vi "Init.vi"(8 "error in (no error)":errorcluster, 11 "reference in":refnum<class "PSU_Keysight_34951A.lvclass">) -> (0 "error out":errorcluster, 3 "reference out":refnum<class "PSU_Keysight_34951A.lvclass">)   [LabVIEW 2022 SP3, in "PSU_Keysight_34951A.lvlib" / "PSU_Keysight_34951A.lvclass"]
uses:
  PSU_Keysight_34951A.lvclass
  Components/PSU_Base.lvlibp/PSU_Base.lvclass
  Components/ViPER.lvlibp/ViPER.lvclass
  C:/Projects/Medulla/ViPER/Examples/Flux_Capacitor_Tester/Components/ViPER.lvlibp/ViPER.lvclass
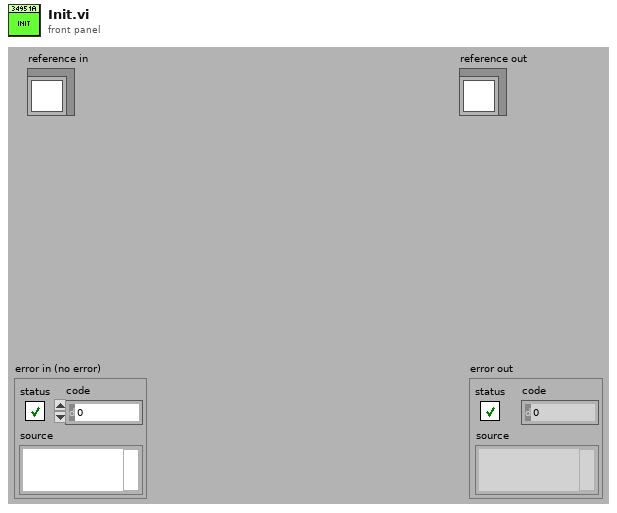
[diagram p1: front panel]
types:
  T1 = typedef "PSU_Keysight_34951A.lvlib/PSU_Keysight_34951A.lvclass/ObjectAttributes.ctl" = cluster{"Config":T2, "VISA res":refnum<visa-resource-name>, "Enabled":bool[], "V":dbl[], "I":dbl[], "Source Type":enum16{"Voltage", "Current"}[]}
  T2 = typedef "PSU_Keysight_34951A.lvlib/PSU_Keysight_34951A.lvclass/Config.ctl" = cluster{"VISA":refnum<visa-resource-name>, "Slot":i32}
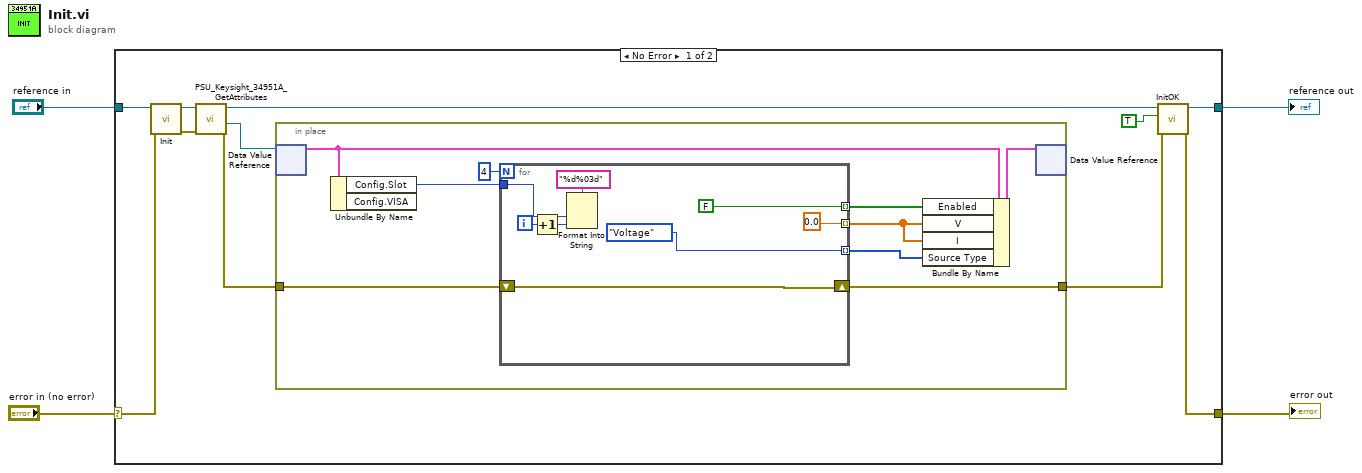
[diagram p0: block diagram]
diagram:
  n1 = case shown="No Error" "error in (no error)" {
    selector: "error in (no error)" -> [w14 w34]
    tunnel: [w5 w34] -> w3
    tunnel: [w8 w33] -> w1
    tunnel: "reference in" -> [w15 w33]
    frame No Error {
      n2 = call-parent "Init.vi"("error in (no error)"=w14, "reference in"=w15) -> ("error out"=w12:errorcluster, "reference out"=w13:refnum<class "PSU_Keysight_34951A.lvclass">)  [unwired: 8 in]
      n3 = call "PSU_Keysight_34951A_GetAttributes.vi"("error in (no error)"=w12, "reference in"=w13) -> ("error out"=w10:errorcluster, "DataRef"=w11:refnum<data-value>, "reference out"=w9:refnum<class "PSU_Keysight_34951A.lvclass">)  [unwired: 6 in, 1 out]
      n4 = in-place {
        in-place-border: w10 -> [w16]
        in-place-border: [w22] -> w6
        n5 = in-place-dvr #1(w11) -> (w24:T1)  [unwired: 1 out]
        n6 = Unbundle By Name(w24) -> ("Config.Slot"=w21:i32)  [unwired: 1 out]
        n7 = for {
          N: 4 -> [_]
          shift-right: [w25] -> w22
          shift-left: w16 -> [w25]
          tunnel: w21 -> [w30]
          tunnel: [FALSE ("Output State (F:Off)")] -> w19 mode=indexing
          tunnel: [0.0 ("Level")] -> w18 mode=indexing
          tunnel: [enum16{"Voltage", "Current"}."Voltage" ("Source Type (0:Voltage)")] -> w17 mode=indexing
          i -> [w31]
          n8 = Increment(x=w31) -> (x+1=w29:i32)
          n9 = Format Into String(format string="%d%03d", w30, w29) -> ()  [unwired: 2 in, 2 out]
        }
        n10 = Bundle By Name(cluster=w24, "Enabled"=w19, "V"=w18, "I"=w18, "Source Type"=w17) -> (w23:T1)
        n11 = in-place-dvr #1(w23) -> ()  [unwired: 2 out]
      }
      n12 = call "InitOK.vi"("error in (no error)"=w6, "Init OK?"=TRUE, "reference in"=w9) -> ("error out"=w5:errorcluster, "reference out"=w8:refnum<class "PSU_Keysight_34951A.lvclass">)  [unwired: 7 in]
    }
    frame Error {
    }
  }
  "error out" <- w3
  "reference out" <- w1
